vi "waitForNewImage.vi"(8 "error in (no error)":errorcluster, 9 "timeout_s":dbl=nan, 10 "delay":bool=TRUE, 11 "Camera in":refnum<class "Camera.lvclass">) -> (0 "error out":errorcluster, 3 "Camera out":refnum<class "Camera.lvclass">)   [LabVIEW 2019, in "Camera.lvclass"]
doc: "Waits for a new image to appear in the recorder memory. In recorder mode 'sequence non\nblocking', 'ring buffer'. and 'fifo', the function record.vi returns immediately.\nTherefore, this function can be used to wait for the next image from the camera before calling\nimage.vi, images.vi, or image_average.vi."
uses:
  Camera.lvclass
  Camera.lvclass/Camera.ctl
  pco.recorder/Recorder.lvlib
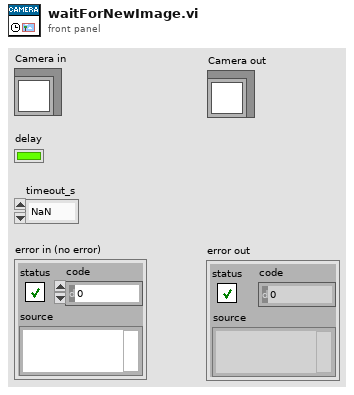
[diagram p1: front panel]
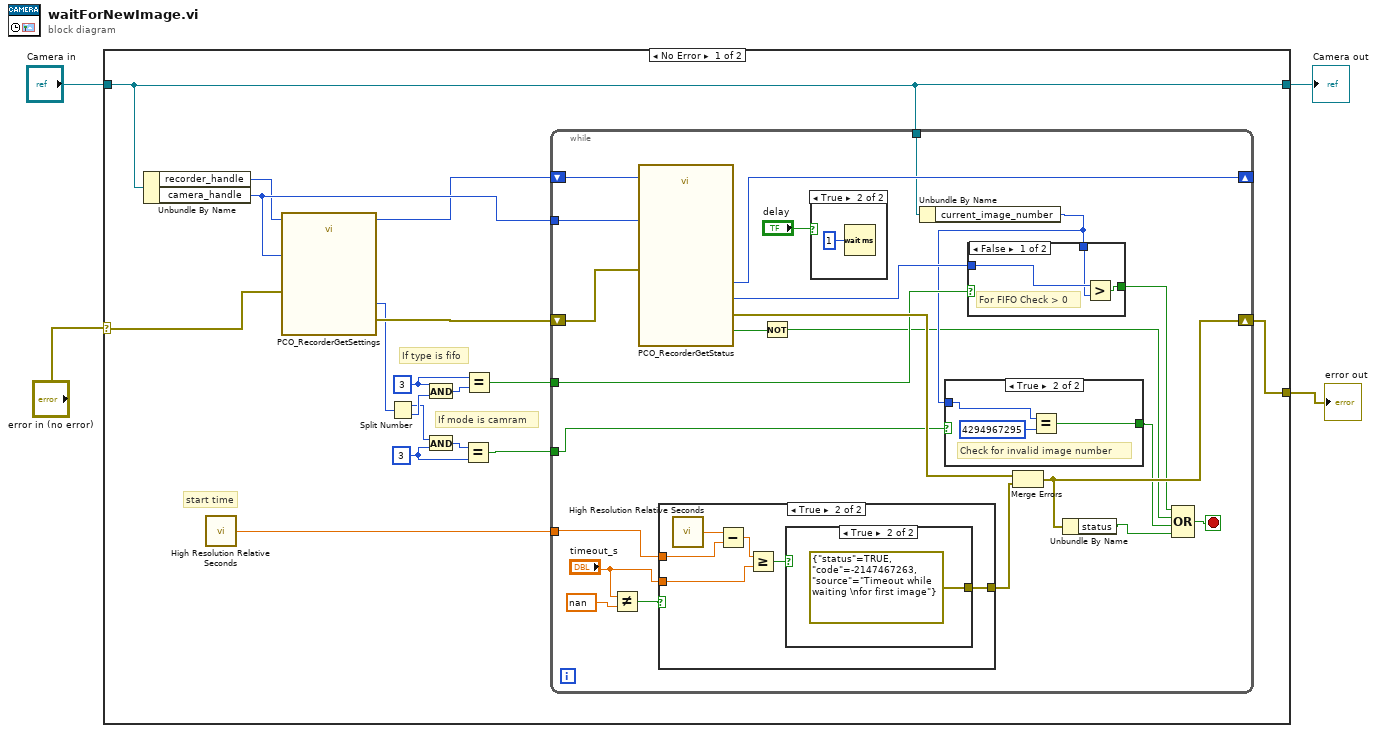
[diagram p0: block diagram]
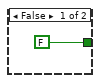
[diagram p2: hidden frame]
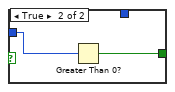
[diagram p3: hidden frame]
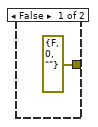
[diagram p4: hidden frame]
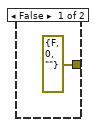
[diagram p5: hidden frame]
diagram:
  n1 = case shown="No Error" "error in (no error)" {
    selector: "error in (no error)" -> [w17 w65]
    tunnel: [w9 w65] -> w2
    tunnel: [w20 w64] -> w1
    tunnel: "Camera in" -> [w20 w64]
    frame No Error {
      w6 = u16 3 ("dwRecMode")
      w11 = u16 3 ("dwRecMode")
      # "If mode is camram"
      # "If type is fifo"
      # "start time"
      n2 = Unbundle By Name(w20) -> ("recorder_handle"=w18:u64, "camera_handle"=w19:u64)
      n3 = call <vilib>:"High Resolution Relative Seconds.vi"() -> ("relative seconds"=w21:dbl)
      n4 = call "PCO_RecorderGetSettings.vi"("phRec"=w18, "phCam"=w19, "error in (no error)"=w17) -> ("phRec out"=w15:u64, "dwRecMode"=w14:u32, "error out"=w16:errorcluster)  [unwired: 4 in, 6 out]
      n5 = Split Number(x=w14) -> (hi(x)=w8:u16, lo(x)=w13:u16)
      n6 = And(x=w11, y=w13) -> (x .and. y?=w12:u16)
      n7 = And(x=w8, y=w6) -> (x .and. y?=w7:u16)
      n8 = Equal?(x=w7, y=w6) -> (x = y?=w5:bool)
      n9 = Equal?(x=w11, y=w12) -> (x = y?=w10:bool)
      n10 = while {
        shift-right: [w34] -> w9
        shift-left: w16 -> [w43]
        shift-right: [w42] -> _
        shift-left: w15 -> [w44]
        tunnel: w19 -> [w41]
        tunnel: w21 -> [w37]
        tunnel: w20 -> [w30]
        tunnel: w10 -> [w29]
        tunnel: w5 -> [w28]
        stop <- w40 stop-if-true
        n11 = Not Equal?(x="timeout_s", y=nan) -> (x != y?=w38:bool)
        n12 = call "PCO_RecorderGetStatus.vi"("phRec"=w44, "phCam"=w41, "error in (no error)"=w43) -> ("dwProcImgCount"=w31:u32, "phRec out"=w42:u64, "bIsRunning"=w23:bool, "error out"=w35:errorcluster)  [unwired: 5 in, 8 out]
        n13 = case shown="True" w38 {
          tunnel: w37 -> [_ w59]
          tunnel: "timeout_s" -> [_ w57]
          tunnel: [errorcluster {"status"=FALSE, "code"=0, "source"=""} ("error constant") w55] -> w36
          frame False {
          }
          frame True {
            n14 = call <vilib>:"High Resolution Relative Seconds.vi"() -> ("relative seconds"=w60:dbl)
            n15 = Subtract(x=w60, y=w59) -> (x-y=w58:dbl)
            n16 = Greater Or Equal?(x=w58, y=w57) -> (x >= y?=w56:bool)
            n17 = case shown="True" w56 {
              tunnel: [errorcluster {"status"=FALSE, "code"=0, "source"=""} ("error constant") errorcluster {"status"=TRUE, "code"=-2147467263, "source"="Timeout while waiting \nfor first image"} ("error constant")] -> w55
              frame False {
              }
              frame True {
              }
            }
          }
        }
        n18 = Not(x=w23) -> (.not. x?=w22:bool)
        n19 = case shown="True" "delay" {
          frame False {
          }
          frame True {
            n20 = Wait (ms)(milliseconds to wait=u32 1) -> ()  [unwired: 1 out]
          }
        }
        n21 = Unbundle By Name(w30) -> ("current_image_number"=w27:u32)
        n22 = case shown="True" w28 {
          tunnel: [FALSE w46] -> w25
          tunnel: w27 -> [_ w47]
          frame False {
          }
          frame True {
            # "Check for invalid image number"
            n23 = Equal?(x=w47, y=u32 4294967295) -> (x = y?=w46:bool)
          }
        }
        n24 = case shown="False" w29 {
          tunnel: [w51 w52] -> w24
          tunnel: w31 -> [w50 w53]
          tunnel: w27 -> [w49 _]
          frame False {
            # "For FIFO Check > 0"
            n25 = Greater?(x=w50, y=w49) -> (0:w51:bool)
          }
          frame True {
            n26 = Greater Than 0?(x=w53) -> (x > 0?=w52:bool)
          }
        }
        n27 = Merge Errors(w35, w36) -> (w34:errorcluster)
        n28 = Unbundle By Name(w34) -> ("status"=w26:bool)
        n29 = Compound Arithmetic op=OR(w24, w22, w25, w26) -> (w40:bool)
      }
    }
    frame Error {
    }
  }
  "error out" <- w2
  "Camera out" <- w1
